vi "Console - Process Strings.vi"(11 "Unprocessed String":string) -> (3 "Processed String":string)   [LabVIEW 2017, in "Communications Console Library.lvlib"]
doc: "Process a multi-line string, removing any blank lines and extra spaces."
uses:
  Communications Console Library.lvlib
  <vilib>/Utility/error.llb/whitespace.ctl
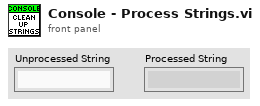
[diagram p1: front panel]
types:
  T1 = typedef "whitespace.ctl" = u16
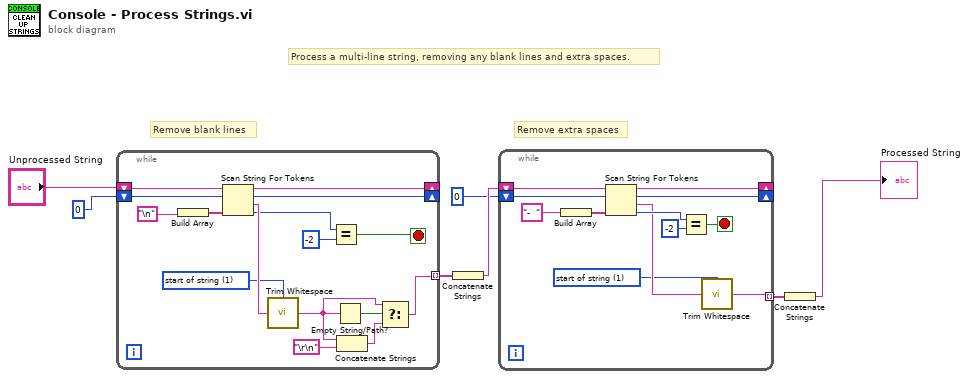
[diagram p0: block diagram]
diagram:
  # "Process a multi-line string, removing any blank lines and extra spaces."
  # "Remove extra spaces"
  # "Remove blank lines"
  n1 = while {
    shift-right: [w22] -> _
    shift-left: "Unprocessed String" -> [w23]
    tunnel: [w13] -> w6 mode=indexing
    shift-right: [w17] -> _
    shift-left: 0 ("offset past token") -> [w19]
    stop <- w18 stop-if-true
    w20 = T1 1 items=["both", "start of string", "end of string"] ("location (both)")
    n2 = Build Array("\n") -> (w9:string[])
    n3 = Scan String For Tokens(6:w9, 8:w19, 9:w23) -> (0:w15:i32, 1:w21:string, 2:w17:i32, 3:w22:string)  [unwired: 3 in]
    n4 = call <vilib>:"Trim Whitespace.vi"("string"=w21, "location (both)"=w20) -> ("trimmed string"=w12:string)
    n5 = Equal?(x=w15, y=-2) -> (x = y?=w18:bool)
    n6 = Empty String/Path?(string/path=w12) -> (empty?=w14:bool)
    n7 = Concatenate Strings(w12, "\r\n") -> (w10:string)
    n8 = Select(t=w12, s=w14, f=w10) -> (s? t:f=w13:string)
  }
  n9 = Concatenate Strings(w6) -> (w5:string)
  n10 = while {
    shift-right: [w33] -> _
    shift-left: w5 -> [w34]
    tunnel: [w27] -> w4 mode=indexing
    shift-right: [w26] -> _
    shift-left: 0 ("offset past token") -> [w25]
    stop <- w30 stop-if-true
    w24 = T1 1 items=["both", "start of string", "end of string"] ("location (both)")
    n11 = Build Array("-  ") -> (w35:string[])
    n12 = Scan String For Tokens(6:w35, 8:w25, 9:w34) -> (0:w31:i32, 1:w28:string, 2:w26:i32, 3:w33:string)  [unwired: 3 in]
    n13 = Equal?(x=w31, y=-2) -> (x = y?=w30:bool)
    n14 = call <vilib>:"Trim Whitespace.vi"("string"=w28, "location (both)"=w24) -> ("trimmed string"=w27:string)
  }
  n15 = Concatenate Strings(w4) -> (→"Processed String":string)
